vi "libssh2_session_get_blocking - invalid session - no error 1097.vi"() -> ()   [LabVIEW 2013, in "libssh2_tests.lvlib"]
uses:
  libssh2_tests.lvlib
  libssh2/Session Refnum.ctl
  libssh2/libssh2_init_default.vi
  <vilib>/Utility/error.llb/General Error Handler.vi
  <vilib>/addons/_JKI Toolkits/Caraya/classes/Assert/Assert.vi
  <vilib>/addons/_JKI Toolkits/Caraya/classes/Assert/Assert Not Error.vi
  <vilib>/addons/_JKI Toolkits/Caraya/classes/Test/Test.lvclass
  libssh2/libssh2.lvlib
panel:
  out "error out":errorcluster
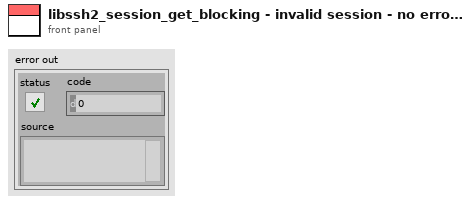
[diagram p1: front panel]
types:
  T1 = typedef "libssh2.lvlib/Session Refnum.ctl" = refnum<k1>
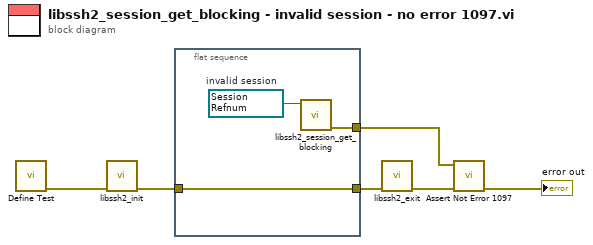
[diagram p0: block diagram]
diagram:
  n1 = call <vilib>:"Define Test.vi"() -> ("error out"=w5:errorcluster)  [unwired: 10 in, 1 out]
  n2 = call-poly "libssh2_init.vi"("error in (no error)"=w5) -> ("error out"=w2:errorcluster)  [unwired: 10 in]
  n3 = flat-sequence {
    tunnel: [w8] -> w3
    tunnel: w2 -> [w8]
    tunnel: [w7] -> w1
    frame #0 {
      w9 = T1 refnum items=["Session"]  # invalid session
      n4 = call "libssh2_session_get_blocking.vi"("session"=w9) -> ("error out"=w7:errorcluster)  [unwired: 9 in, 1 out]
    }
  }
  n5 = call "libssh2_exit.vi"("error in (no error)"=w3) -> ("error out"=w4:errorcluster)  [unwired: 10 in]
  n6 = call "Assert Not Error 1097.vi"("error in (no error)"=w4, "actual value"=w1) -> ("error out"=→"error out":errorcluster)  [unwired: 9 in]
